vi "Configure GPIO.vi"(0 "VISA resource name":refnum<visa-resource-name>, 5 "Enable GPIO Pin (Disabled)":bool[](array[boolean]), 7 "Enable GPIO Output (Disabled)":bool[](array[boolean]), 9 "GPIO Value (Low)":bool[](array[boolean]), 11 "error in (no error)":errorcluster) -> (4 "VISA resource name out":refnum<visa-resource-name>, 15 "error out":errorcluster)   [LabVIEW 2018, in "Ocean Optics 2000 4000.lvlib"]
doc: "Configures the GPIO (General Purpose I/O) pins on the spectrometer. \n\n<b>Note:</b>\n-HR2000 & USB2000 does not have GPIO pins\n-USB2000+ & USB4000 have 8 GPIO pins\n-HR2000+ & HR4000 have 10 GPIO pins"
uses:
  Ocean Optics 2000 4000.lvlib
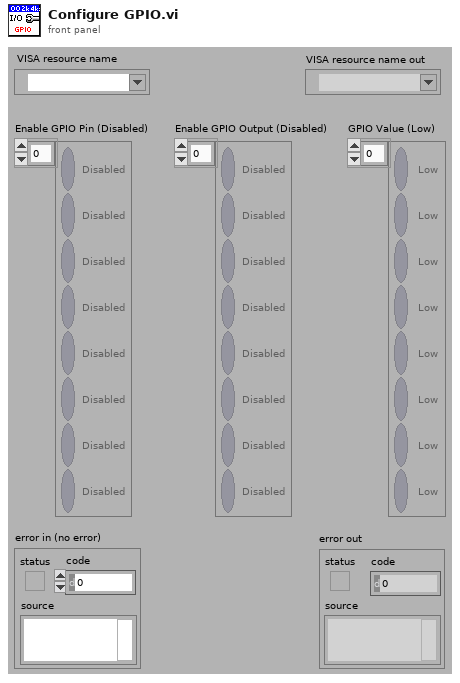
[diagram p1: front panel]
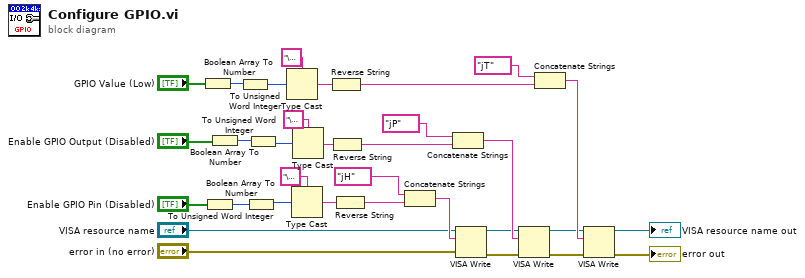
[diagram p0: block diagram]
diagram:
  n1 = Boolean Array To Number(Boolean array="GPIO Value (Low)") -> (number=w24:u32)
  n2 = Boolean Array To Number(Boolean array="Enable GPIO Pin (Disabled)") -> (number=w26:u32)
  n3 = Boolean Array To Number(Boolean array="Enable GPIO Output (Disabled)") -> (number=w25:u32)
  n4 = To Unsigned Word Integer(number=w24) -> (unsigned 16bit integer=w21:u16)
  n5 = To Unsigned Word Integer(number=w26) -> (unsigned 16bit integer=w23:u16)
  n6 = To Unsigned Word Integer(number=w25) -> (unsigned 16bit integer=w22:u16)
  n7 = Type Cast(type="\u0000", x=w21) -> (*(type *) &x=w16:string)
  n8 = Type Cast(type="\u0000", x=w23) -> (*(type *) &x=w17:string)
  n9 = Type Cast(type="\u0000", x=w22) -> (*(type *) &x=w15:string)
  n10 = Reverse String(1:w16) -> (0:w12:string)
  n11 = Reverse String(1:w15) -> (0:w13:string)
  n12 = Reverse String(1:w17) -> (0:w14:string)
  n13 = Concatenate Strings("jH" ("string"), w14) -> (w30:string)
  n14 = Concatenate Strings("jP" ("string"), w13) -> (w31:string)
  n15 = VISA Write(VISA resource name="VISA resource name", write buffer=w30, error in (no error)="error in (no error)") -> (VISA resource name out=w6:refnum<visa-resource-name>, error out=w5:errorcluster)  [unwired: 1 out]
  n16 = VISA Write(VISA resource name=w6, write buffer=w31, error in (no error)=w5) -> (VISA resource name out=w4:refnum<visa-resource-name>, error out=w3:errorcluster)  [unwired: 1 out]
  n17 = Concatenate Strings("jT" ("string"), w12) -> (w32:string)
  n18 = VISA Write(VISA resource name=w4, write buffer=w32, error in (no error)=w3) -> (VISA resource name out=→"VISA resource name out":refnum<visa-resource-name>, error out=→"error out":errorcluster)  [unwired: 1 out]
